vi "Drive System.vi"   [LabVIEW 2018]
uses:
  <vilib>/Rock Robotics/WPI/Utilities/WPI_GetSetVariantRefNum.vi
types:
  T1 = typedef "WPI_JoystickDevRef.ctl" = cluster{"Device":T2}
  T2 = typedef "WPI_JoystickDeviceEnum.ctl" = enum16{"USB 0", "USB 1", "USB 2", "USB 3", "USB 4", "USB 5"}
  T3 = typedef "WPI_MotorControlDeviceRef.ctl" = cluster{"DeviceStatus":errorcluster, "Type":T4, "PWM":cluster{"PWM Channel":T5, "DeadBand":T6}, "CAN":cluster{"Device Number":u8, "SetOutput VI Ref":variant, "GetOutput VI Ref":variant, "Enable VI Ref":variant, "Disable VI Ref":variant, "Data":variant}, "Invert":bool, "DIO PWM":cluster{"PWM \"Enable\" Channel":T5, "DIOChannel":T7, "PWM Rate":dbl}}
  T4 = typedef "WPI_MotorControlType.ctl" = enum16{"PWM", "CAN", "DIO PWM"}
  T5 = typedef "FPGA_DIOPWMChannel.ctl" = enum8{"PWM 0", "PWM 1", "PWM 2", "PWM 3", "PWM 4", "PWM 5", "PWM 6", "PWM 7", "PWM 8", "PWM 9", "PWM MXP 0", "PWM MXP 1", "PWM MXP 2", "PWM MXP 3", "PWM MXP 4", "PWM MXP 5", "PWM MXP 6", "PWM MXP 7", "PWM MXP 8", "PWM MXP 9", "Invalid"}
  T6 = typedef "WPI_PWMDeadband.ctl" = cluster{"Name":string, "maxPositivePwm":i32, "minPositivePwm":i32, "centerPwm":i32, "maxNegativePwm":i32, "minNegativePwm":i32, "angularRange":u16}
  T7 = typedef "FPGA_DIOChannel.ctl" = enum8{"DIO 0", "DIO 1", "DIO 2", "DIO 3", "DIO 4", "DIO 5", "DIO 6", "DIO 7", "DIO 8", "DIO 9", "DIO MXP 0", "DIO MXP 1", "DIO MXP 2", "DIO MXP 3", "DIO MXP 4", "DIO MXP 5", "DIO MXP 6", "DIO MXP 7", "DIO MXP 8", "DIO MXP 9", "DIO MXP 10", "DIO MXP 11", "DIO MXP 12", "DIO MXP 13", "DIO MXP 14", "DIO MXP 15", "SPI Port CS1", "SPI Port CS2", "SPI Port CS3", "SPI Port MISO", "SPI Port MOSI", "Invalid"}
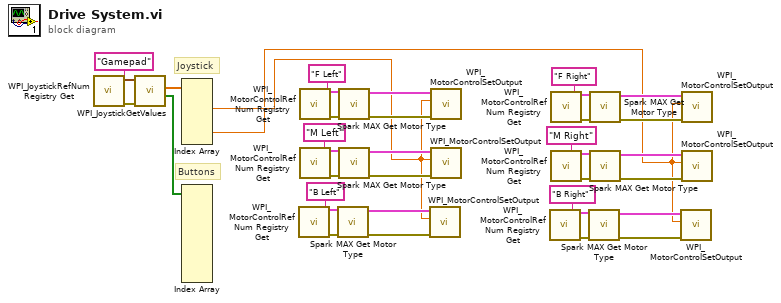
[diagram p0: block diagram]
diagram:
  # "Buttons"
  # "Joystick"
  n1 = call <vilib>:"WPI_JoystickRefNum Registry Get.vi"("refnum name"="Gamepad") -> ("error out"=w37:errorcluster, "JoystickDevRef"=w36:T1)  [unwired: 9 in]
  n2 = call <vilib>:"WPI_JoystickGetValues.vi"("error in (no error)"=w37, "JoystickDevRef"=w36) -> ("Buttons"=w34:bool[], "Axes"=w35:dbl[])  [unwired: 5 in, 3 out]
  n3 = Index Array(array=w35) -> (element #2=w18:dbl, element #5=w2:dbl)  [unwired: 6 in, 4 out]
  n4 = Index Array(array=w34) -> ()  [unwired: 10 in, 10 out]
  n5 = call <vilib>:"WPI_MotorControlRefNum Registry Get.vi"("refnum name"="B Left") -> ("error out"=w22:errorcluster, "MotorControlDevRef"=w21:T3)  [unwired: 9 in]
  n6 = call <vilib>:"WPI_MotorControlRefNum Registry Get.vi"("refnum name"="F Left") -> ("error out"=w32:errorcluster, "MotorControlDevRef"=w31:T3)  [unwired: 9 in]
  n7 = call <vilib>:"WPI_MotorControlRefNum Registry Get.vi"("refnum name"="M Left") -> ("error out"=w27:errorcluster, "MotorControlDevRef"=w26:T3)  [unwired: 9 in]
  n8 = call <vilib>:"Spark MAX Get Motor Type.vi"("error in (no error)"=w22, "MotorControlDeviceRef in"=w21) -> ("error out"=w20:errorcluster, "MotorControlDeviceRef out"=w19:T3)  [unwired: 7 in, 1 out]
  n9 = call <vilib>:"Spark MAX Get Motor Type.vi"("error in (no error)"=w32, "MotorControlDeviceRef in"=w31) -> ("error out"=w30:errorcluster, "MotorControlDeviceRef out"=w29:T3)  [unwired: 7 in, 1 out]
  n10 = call <vilib>:"Spark MAX Get Motor Type.vi"("error in (no error)"=w27, "MotorControlDeviceRef in"=w26) -> ("error out"=w25:errorcluster, "MotorControlDeviceRef out"=w24:T3)  [unwired: 7 in, 1 out]
  n11 = call <vilib>:"WPI_MotorControlSetOutput.vi"("error in (no error)"=w20, "Output"=w18, "MotorControlDevRef"=w19) -> ()  [unwired: 6 in, 3 out]
  n12 = call <vilib>:"WPI_MotorControlSetOutput.vi"("error in (no error)"=w30, "Output"=w18, "MotorControlDevRef"=w29) -> ()  [unwired: 6 in, 3 out]
  n13 = call <vilib>:"WPI_MotorControlSetOutput.vi"("error in (no error)"=w25, "Output"=w18, "MotorControlDevRef"=w24) -> ()  [unwired: 6 in, 3 out]
  n14 = call <vilib>:"WPI_MotorControlRefNum Registry Get.vi"("refnum name"="B Right") -> ("error out"=w6:errorcluster, "MotorControlDevRef"=w5:T3)  [unwired: 9 in]
  n15 = call <vilib>:"WPI_MotorControlRefNum Registry Get.vi"("refnum name"="F Right") -> ("error out"=w16:errorcluster, "MotorControlDevRef"=w15:T3)  [unwired: 9 in]
  n16 = call <vilib>:"WPI_MotorControlRefNum Registry Get.vi"("refnum name"="M Right") -> ("error out"=w11:errorcluster, "MotorControlDevRef"=w10:T3)  [unwired: 9 in]
  n17 = call <vilib>:"Spark MAX Get Motor Type.vi"("error in (no error)"=w6, "MotorControlDeviceRef in"=w5) -> ("error out"=w4:errorcluster, "MotorControlDeviceRef out"=w3:T3)  [unwired: 7 in, 1 out]
  n18 = call <vilib>:"Spark MAX Get Motor Type.vi"("error in (no error)"=w16, "MotorControlDeviceRef in"=w15) -> ("error out"=w14:errorcluster, "MotorControlDeviceRef out"=w13:T3)  [unwired: 7 in, 1 out]
  n19 = call <vilib>:"Spark MAX Get Motor Type.vi"("error in (no error)"=w11, "MotorControlDeviceRef in"=w10) -> ("error out"=w9:errorcluster, "MotorControlDeviceRef out"=w8:T3)  [unwired: 7 in, 1 out]
  n20 = call <vilib>:"WPI_MotorControlSetOutput.vi"("error in (no error)"=w4, "Output"=w2, "MotorControlDevRef"=w3) -> ()  [unwired: 6 in, 3 out]
  n21 = call <vilib>:"WPI_MotorControlSetOutput.vi"("error in (no error)"=w14, "Output"=w2, "MotorControlDevRef"=w13) -> ()  [unwired: 6 in, 3 out]
  n22 = call <vilib>:"WPI_MotorControlSetOutput.vi"("error in (no error)"=w9, "Output"=w2, "MotorControlDevRef"=w8) -> ()  [unwired: 6 in, 3 out]
